vi "Send commands to tool.vi"(1 "Tool command":T1, 7 "Input Data":dbl, 11 "error in":errorcluster) -> (8 "OK":bool, 15 "error out":errorcluster)   [LabVIEW 2011]
uses:
  Stroker/def/Tool specific commands.ctl
  List of nodes in tool.ctl
  List of tools.ctl
  Variable List Tool Analog.ctl
  GUI/Controls/Slips Type Radio.ctl
  Application Structure/Loop ID.ctl
  emi Lib/System 01/0 - General/App/Loop control 2/Private/_emi_SMLoop Control Single.vi
  emi Lib/System 01/0 - General/App/Loop control/Private/_emi_GFV Loop Enable.vi
  emi Lib/System 01/0 - General/App/Loop control/Private/_emi_GFV Loop Linking.vi
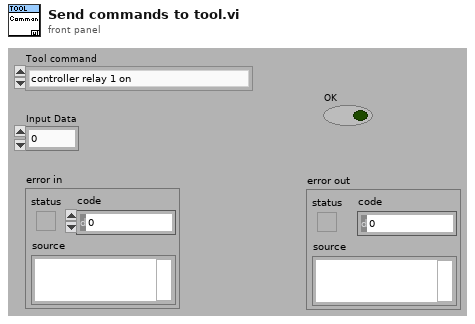
[diagram p1: front panel]
types:
  T1 = typedef "Tool specific commands.ctl" = enum16{"controller relay 1 on", "controller relay 1 off", "controller relay 2 on", "controller relay 2 off", "Solonoid 1 (master) on", "Solonoid 1 (master) off", "Solonoid 2 (Stroker) on", "Solonoid 2 (Stroker) off", "Solonoid 3 (Anchor) on", "Solonoid 3 (Anchor) off", "Controller relay 1 & 2 on", "Controller relay 1 & 2 off", "Controller relay 1 on, 2 off", "Controller relay 1 off, 2 on", "STROKER tool: Stop Force Mon", "High-G Stop", "High-G Get data", "High-G Stop Get data", "STROKER tool: Stroke out", "STROKER tool: Stroke in", "STROKER tool: Stroke stop", "STROKER tool: Stroke go to", "STROKER tool: Stop Homing", "STROKER tool: Start Force Mon dir in", "STROKER tool: Start Force Mon dir out", "Controller STOP"}
  T2 = typedef "List of tools.ctl" = enum16{"Stroker", "Driller", "Tractor"}
  T3 = typedef "Options  All pages and custom.ctl" = cluster{"P 1 (App)":T4, "P 2":T5, "P 3":T6, "P 4":T9, "P 5":T14, "P 6 (Err)":T15, "P 7 (Expert)":T16, "P 8 (Depth)":T18, "C 1":T19, "C 2":T20}
  T4 = typedef "Options Page 1 (App).ctl" = cluster{"Result files":path, "PCP Interface":string, "Tractor/Stroker Interface":string, "Tractor Interface":string, "Modem Status Interface":string, "Audible Alarm":bool, "Force alarm on Technical":bool, "Force alarm on HH":bool, "Force alarm on LL":bool, "Force alarm on H":bool, "Force alarm on L":bool}
  T5 = typedef "Options Page 2.ctl" = cluster{"Solenoid & Relay latching time":u16, "Tractor relay 1":dbl, "Tractor relay 2":dbl, "Tractor Solenoid limit":dbl}
  T6 = typedef "Options Page 3.ctl" = cluster{"Min resistance":dbl, "Max resistance":dbl, "Head voltage range":T7, "Max voltage jump":dbl, "Maximum resistance change":dbl, "Start Telemetry Voltage":dbl, "Start Telemetry Timeout":dbl, "Start Motor Voltage":dbl, "Stop Motor Voltage":dbl, "Pass Mode Warning Voltage":dbl, "Relay Switch Voltage":dbl, "Relay Status Loss Voltage":dbl, "Samples to average":i32, "PSU type DO NOT USE":T8, "Magna OVP":dbl, "Magna Current Limit":dbl}
  T7 = typedef "PCP type List.ctl" = enum16{"0 - 350V", "0 - 450V", "0 - 600V"}
  T8 = typedef "PSU Type.ctl" = enum16{"Unipower", "Magna 8.3A", "Magna 12A", "None"}
  T9 = typedef "Options Page 4.ctl" = cluster{"Solenoid & Relay latching time":u16, "Stroker relay 1":dbl, "Stroker Relay 2":dbl, "Stroker Solenoid limit":dbl, "Force det.":T10, "Stroke force lim.":dbl, "Anchor Enabled Pressure":dbl, "Tacometer puls":dbl, "Default anchor behavior":T11, "Default stroker behavior":T12, "Default stroker force limit (tonne)":dbl, "Slips Size":T13}
  T10 = typedef "Stroke force selector.ctl" = enum16{"Stroke in = node 1", "Strok out = node 1"}
  T11 = typedef "Default anchor behavior.ctl" = enum16{"Do nothing", "Set Anchor", "Release Anchor"}
  T12 = typedef "Default stroker behavior.ctl" = enum16{"Do nothing", "Stop", "Go Out", "Go In"}
  T13 = typedef "Slips Type Radio.ctl" = enum32{"No Selection", "338 MRS", "3,9 MRS"}
  T14 = typedef "Options Page 5.ctl" = cluster{"Solenoid & Relay latching time":u16, "Driller relay 1":dbl, "Driller Relay 2":dbl, "Driller  Solenoid limit":dbl}
  T15 = typedef "Options Page 6 (Err).ctl" = cluster{"Error and event files":path}
  T16 = typedef "Options Page 7 (Expert).ctl" = cluster{"Show Debug":bool, "Log debug messages":bool, "Additional debug messages":bool, "Start Beagle with Simulator data":bool, "Workshop mode":bool, "Modem baud":u16, "enumCANCOM":bool, "Modem sim":T17, "Telemetry Timeout Disable":i32, "Buffer size":i32, "Upd regular data":bool, "Cable comp":cluster{"VMOD1 Voltage(V)":dbl, "VMOD2 Voltage(V)":dbl}}
  T17 = typedef "Modem simulation setup.ctl" = cluster{"Modem dealay sim":bool, "Sim baud Tx":u16, "Bit Error fraction Tx":dbl, "Sim baud Rx":u16, "Bit Error fraction Rx":dbl}
  T18 = typedef "Options Page 8 (Depth).ctl" = cluster{"Winch Spool Circumference":dbl, "Winch Pulses per Revolution":dbl, "Current Depth":dbl}
  T19 = typedef "Options Custom 1.ctl" = cluster{"Depth Updated":bool, "Depth Offset":dbl}
  T20 = typedef "Options Custom 2.ctl" = cluster{"Placeholder":bool}
  T21 = typedef "Variable List Tool Analog.ctl" = enum16{"Tool Max Temperature", "Tool (Controller) Temperature", "Tool Supply Voltage", "Tool (Controller) Current", "Tool Acceleration X", "Tool Acceleration Y", "Tool Acceleration Z", "Tool Acceleration Sum", "Tool Inclination", "Tool Rotation", "Tool GP Sensor 1", "Tool GP Sensor 2", "Tool (Pressure 1) Temperature", "Tool Pressure 1 RAW", "Tool (Pressure 2) Temperature", "Tool Pressure 2 RAW", "Tool (Solenoid) Temperature", "Tool Solenoid Position", "PSU Temp", "Head Voltage", "PSU Main Voltage out", "PSU Main Current out", "Upper Tension Sub Temp", "Tool Upper Tension Sub Raw", "Lower Tension Sub Temp", "Tool Lower Tension Sub Raw", "Tool Var27 - Reserved", "Tool Var28 - Reserved", "Tool Var29 - Reserved", "Tool Var30 - Reserved", "Stroke Extension", "Stroke In Force", "Stroke Out Force", "Stroke Force", "Stroker Pressure 1", "Stroker Pressure 2", "Stroker Upper Tension Sub", "Stroker Lower Tension Sub", "Stroker Var09 - Reserved", "Stroker Var10 - Reserved", "Tractor Upper Tension Sub", "Tractor Lower Tension Sub", "Tractor Var03 - Reserved", "Tractor Var04 - Reserved", "Tool Temperature sensor", "Tool Motor Voltage", "Tool Motor Current", "Tool Motor Torque", "Tool weight on bit", "Tool Motor RPM"}
  T22 = typedef "Loop ID.ctl" = enum16{"Main-QSM", "Main-Dialog", "Main-Ind Upd", "Main-Graph Upd", "Main-Debug", "Main-DebugW1", "Main-DebugW2", "Main-SE Handler", "Interface-PCP", "Interface-CANbus", "Interface-Modem", "Var Handling-Beat", "Var Handling-From PCP", "Var Handling-File storage", "Var Handling-From Simulator", "GUI-GrphW Mast", "GUI-GrphW Slav", "SIM-Tool W1", "SIM-Tool W2", "Alm-Sound", "LEIN-motor", "Tool data gatherer Qer", "Tool Data LEIN STAT2 dekoder", "Indicator Value Update", "Tool STAT2 dedicated reader", "Tool ID handler", "Detail View L1", "Detail View L2", "Main display enable view", "Sequence runner", "Voltage setpoint", "Resistance setpoint", "Stroker Wizard L1", "Stroker Wizard L2", "Alarm Handling", "Annotations Tip Strip", "Magna Interface", "Modem Status", "Var Handling - Modem Status", "Power interface detector"}
  T23 = typedef "LEIN custom reply Q.ctl" = refnum<queue>
  T24 = typedef "List of nodes in tool.ctl" = u16
  T25 = typedef "User Setting Analog Channel Bg.ctl" = cluster{"Scaling":T26, "Limits and responces":T27, "Allow Graph selection by user":bool, "Unit":u16}
  T26 = typedef "Scaling.ctl" = cluster{"Gain":dbl, "Offset":dbl}
  T27 = typedef "Alarm Setup Analog.ctl" = cluster{"Technical Error(NA)":T28, "LL":T28, "L":T28, "H":T28, "HH":T28, "Limits":T30}
  T28 = typedef "Alarm Responce.ctl" = cluster{"Action":T29, "Alarm":bool}
  T29 = typedef "Action List.ctl" = enum16{"No Action", "Stop Motor", "Turn Off HV"}
  T30 = typedef "Limits.ctl" = cluster{"LL":dbl, "L":dbl, "H":dbl, "HH":dbl}
  T31 = typedef "LEIN Reply Holder.ctl" = cluster{"Reply msg(cmdif no reply)":T32, "Reply time":timestamp, "Valid reply":bool}
  T32 = typedef "LEIN CMD Cluster.ctl" = cluster{"SID":u8, "ANF":bool, "CMD":T33, "DATA":u8[]}
  T33 = typedef "LEIN CMD List.ctl" = enum8{"ACTI", "TASK", "RES0", "STAT", "RES1", "RES2", "RES3", "USER"}
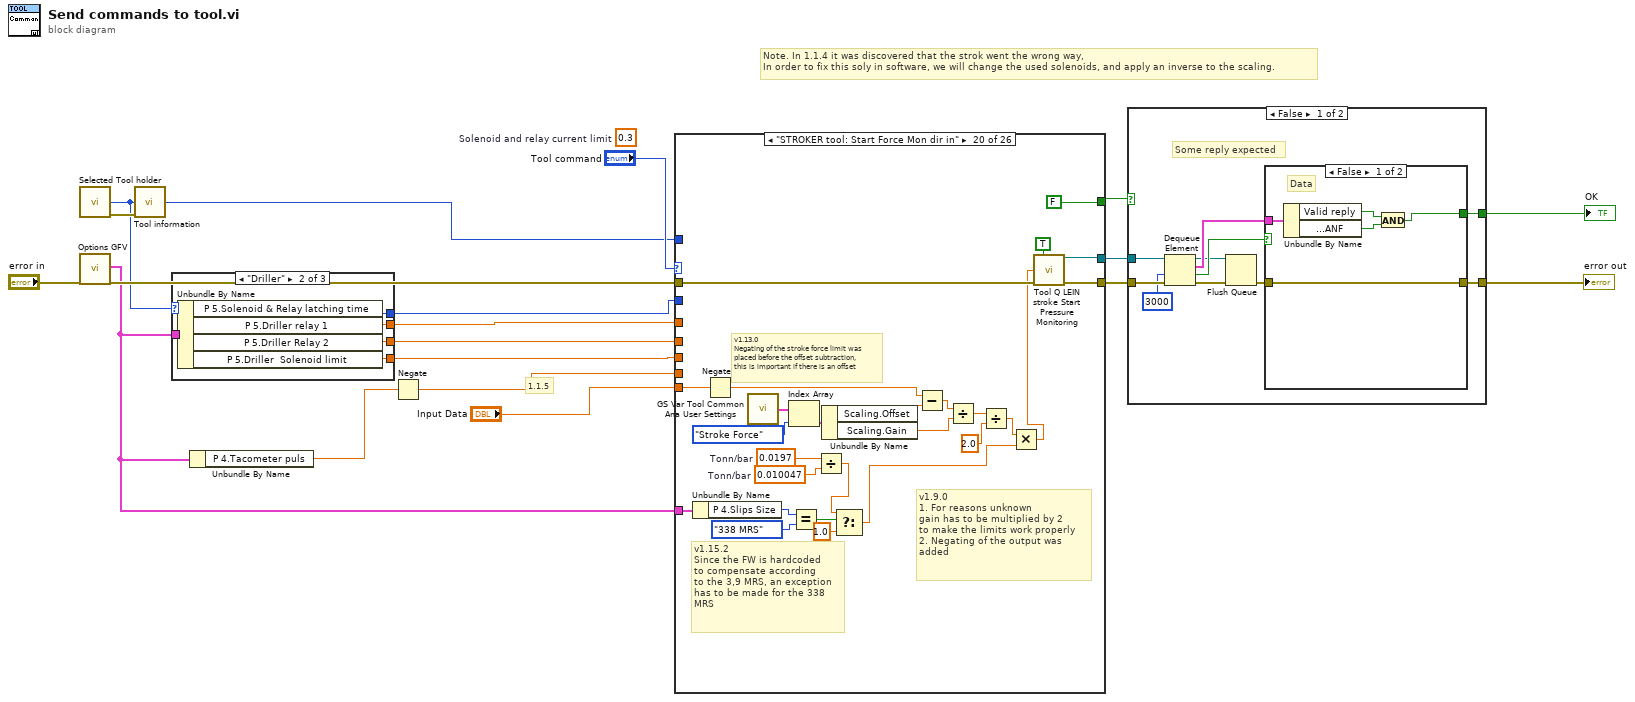
[diagram p0: block diagram]
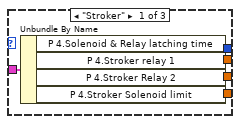
[diagram p2: hidden frame]
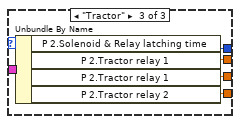
[diagram p3: hidden frame]
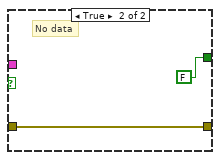
[diagram p4: hidden frame]
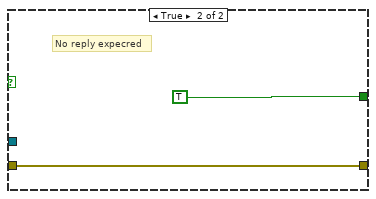
[diagram p5: hidden frame]
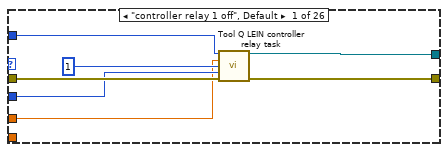
[diagram p6: hidden frame]
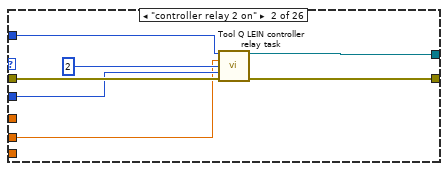
[diagram p7: hidden frame]
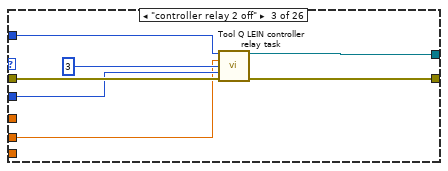
[diagram p8: hidden frame]
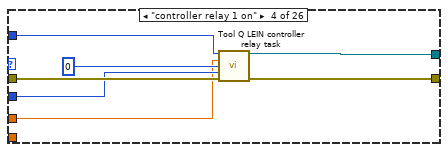
[diagram p9: hidden frame]
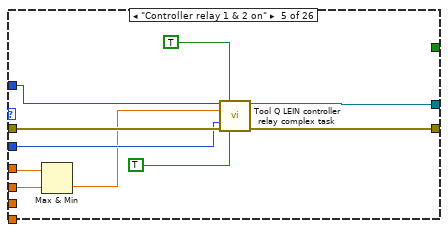
[diagram p10: hidden frame]
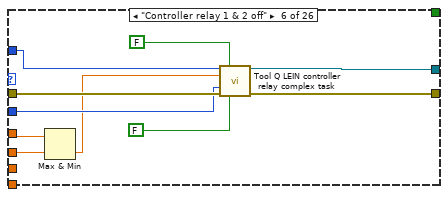
[diagram p11: hidden frame]
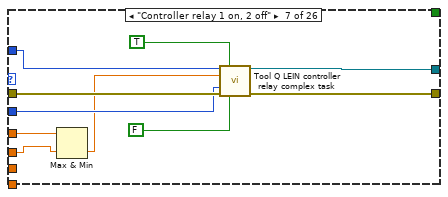
[diagram p12: hidden frame]
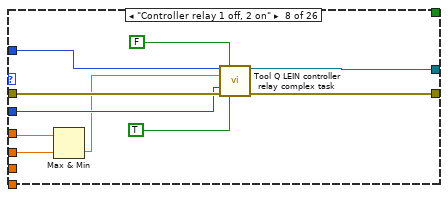
[diagram p13: hidden frame]
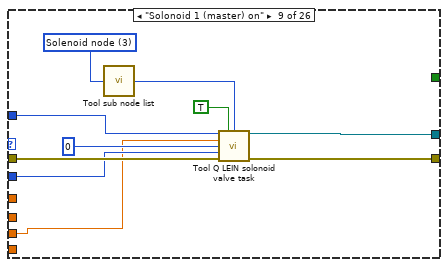
[diagram p14: hidden frame]
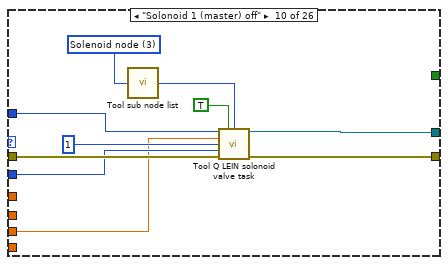
[diagram p15: hidden frame]
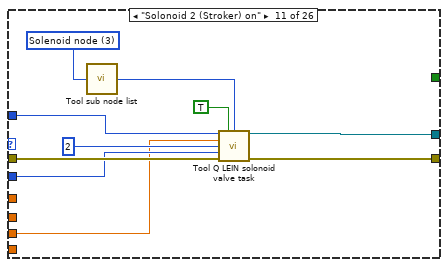
[diagram p16: hidden frame]
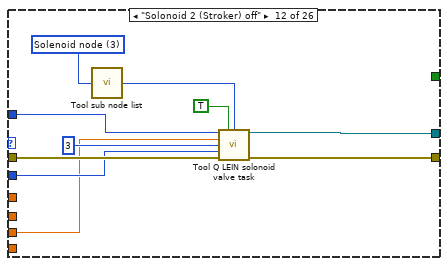
[diagram p17: hidden frame]
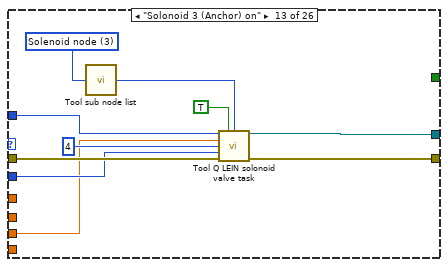
[diagram p18: hidden frame]
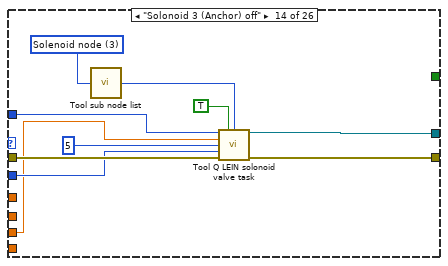
[diagram p19: hidden frame]
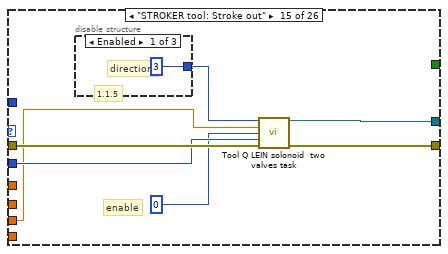
[diagram p20: hidden frame]
diagram:
  (unwired) 0.3  # Solenoid and relay current limit
  # "1.1.5"
  # "Note. In 1.1.4 it was discovered that the strok went the wrong way,\nIn order to fix this soly in software, we will change the used solenoids, and apply an inverse to the scaling."
  n1 = call "Selected Tool holder.vi"() -> ("Tool out"=w3:T2, "error out"=w6:errorcluster)  [unwired: 14 in]
  n2 = call "Options GFV.vi"("error in (no error)"="error in") -> ("Options"=w2:T3, "error out"=w11:errorcluster)  [unwired: 16 in, 1 out]
  n3 = call "Tool information.vi"("Tool in"=w3, "error in (no error)"=w6) -> ("Main node address"=w4:u8)  [unwired: 10 in, 3 out]
  n4 = case shown="\"Driller\"" w3 {
    tunnel: [w24 w29 w34] -> w10
    tunnel: [w23 w28 w33] -> w9
    tunnel: [w22 w27 w32] -> w8
    tunnel: w2 -> [w21 w26 w31]
    tunnel: [w20 w25 w30] -> w1
    frame "Stroker" {
      n5 = Unbundle By Name(w21) -> ("P 4.Solenoid & Relay latching time"=w20:u16, "P 4.Stroker relay 1"=w24:dbl, "P 4.Stroker Relay 2"=w23:dbl, "P 4.Stroker Solenoid limit"=w22:dbl)
    }
    frame "Driller" {
      n6 = Unbundle By Name(w26) -> ("P 5.Solenoid & Relay latching time"=w25:u16, "P 5.Driller relay 1"=w29:dbl, "P 5.Driller Relay 2"=w28:dbl, "P 5.Driller  Solenoid limit"=w27:dbl)
    }
    frame "Tractor" {
      n7 = Unbundle By Name(w31) -> ("P 2.Solenoid & Relay latching time"=w30:u16, "P 2.Tractor relay 1"=w34:dbl, "P 2.Tractor relay 1"=w33:dbl, "P 2.Tractor relay 2"=w32:dbl)
    }
  }
  n8 = Unbundle By Name(w2) -> ("P 4.Tacometer puls"=w5:dbl)
  n9 = Negate(x=w5) -> (-x=w7:dbl)
  n10 = case shown="\"STROKER tool: Start Force Mon dir in\"" "Tool command" {
    tunnel: [w40 w47 w54 w61 w70 w80 w90 w100 w111 w121 w131 w141 w151 w161 w169 w178 w187 w207 w212 w237 w261 w267 w281 w285 w290 w295] -> w16
    tunnel: w11 -> [w41 w48 w55 w62 w72 w82 w92 w102 w112 w122 w132 w142 w152 w162 w168 w177 w189 w208 w213 w238 w262 w268 w282 w286 w291 w296]
    tunnel: w1 -> [w39 w46 w53 w60 w71 w81 w91 w101 w110 w120 w130 w140 w150 w160 w167 w176 w188 w206 _ _ _ _ _ _ _ _]
    tunnel: "Input Data" -> [_ _ _ _ _ _ _ _ _ _ _ _ _ _ _ _ _ w196 _ w226 w254 _ _ _ _ _]
    tunnel: [w37 w44 w51 w58 w67 w77 w87 w97 w108 w118 w128 w138 w148 w158 w164 w173 w185 w205 w210 w235 w260 w266 w280 _ _ w294] -> w15
    tunnel: [_ _ _ _ _ _ _ _ _ _ _ _ _ _ _ _ _ _ FALSE FALSE FALSE _ _ TRUE TRUE _] -> w17
    tunnel: w10 -> [w36 _ _ w57 w65 w75 w86 w95 _ _ _ _ _ _ _ _ _ _ _ _ _ _ _ _ _ _]
    tunnel: w9 -> [_ w43 w50 _ w66 w76 w85 w96 _ _ _ _ _ _ _ _ _ _ _ _ _ _ _ _ _ _]
    tunnel: w8 -> [_ _ _ _ _ _ _ _ w106 w116 w126 w136 w146 w156 w163 w172 w184 w203 _ _ _ _ _ _ _ _]
    tunnel: w7 -> [_ _ _ _ _ _ _ _ _ _ _ _ _ _ _ _ _ w201 _ _ _ _ _ _ _ _]
    tunnel: w4 -> [w35 w42 w49 w56 w63 w73 w83 w93 w105 w115 w125 w135 w143 w155 _ _ _ _ _ _ _ w265 w279 _ _ w293]
    tunnel: w2 -> [_ _ _ _ _ _ _ _ _ _ _ _ _ _ _ _ _ _ _ w224 w243 _ _ _ _ _]
    frame "controller relay 1 off", Default {
      n11 = call "Tool Q LEIN controller relay task.vi"("Controller addres"=w35, "current limit(0.2A)"=w36, "outpuyt channel"=u8 1, "time (50 ms)"=w39, "error in (no error)"=w41) -> ("LEIN custom reply Q"=w37:T23, "error out"=w40:errorcluster)  [unwired: 9 in]
    }
    frame "controller relay 2 on" {
      n12 = call "Tool Q LEIN controller relay task.vi"("Controller addres"=w42, "current limit(0.2A)"=w43, "outpuyt channel"=u8 2, "time (50 ms)"=w46, "error in (no error)"=w48) -> ("LEIN custom reply Q"=w44:T23, "error out"=w47:errorcluster)  [unwired: 9 in]
    }
    frame "controller relay 2 off" {
      n13 = call "Tool Q LEIN controller relay task.vi"("Controller addres"=w49, "current limit(0.2A)"=w50, "outpuyt channel"=u8 3, "time (50 ms)"=w53, "error in (no error)"=w55) -> ("LEIN custom reply Q"=w51:T23, "error out"=w54:errorcluster)  [unwired: 9 in]
    }
    frame "controller relay 1 on" {
      n14 = call "Tool Q LEIN controller relay task.vi"("Controller addres"=w56, "current limit(0.2A)"=w57, "outpuyt channel"=u8 0, "time (50 ms)"=w60, "error in (no error)"=w62) -> ("LEIN custom reply Q"=w58:T23, "error out"=w61:errorcluster)  [unwired: 9 in]
    }
    frame "Controller relay 1 & 2 on" {
      n15 = Max & Min(x=w65, y=w66) -> (min(x,y)=w64:dbl)  [unwired: 1 out]
      n16 = call "Tool Q LEIN controller relay complex task.vi"("Controller ID"=w63, "Relay 1 close(on)"=TRUE, "current limit(0.2A)"=w64, "time (50 ms)"=w71, "error in (no error)"=w72, "Relay 2 close(on)"=TRUE) -> ("LEIN custom reply Q"=w67:T23, "error out"=w70:errorcluster)  [unwired: 8 in]
    }
    frame "Controller relay 1 & 2 off" {
      n17 = Max & Min(x=w75, y=w76) -> (min(x,y)=w74:dbl)  [unwired: 1 out]
      n18 = call "Tool Q LEIN controller relay complex task.vi"("Controller ID"=w73, "Relay 1 close(on)"=FALSE, "current limit(0.2A)"=w74, "time (50 ms)"=w81, "error in (no error)"=w82, "Relay 2 close(on)"=FALSE) -> ("LEIN custom reply Q"=w77:T23, "error out"=w80:errorcluster)  [unwired: 8 in]
    }
    frame "Controller relay 1 on, 2 off" {
      n19 = Max & Min(x=w86, y=w85) -> (min(x,y)=w84:dbl)  [unwired: 1 out]
      n20 = call "Tool Q LEIN controller relay complex task.vi"("Controller ID"=w83, "Relay 1 close(on)"=TRUE, "current limit(0.2A)"=w84, "time (50 ms)"=w91, "error in (no error)"=w92, "Relay 2 close(on)"=FALSE) -> ("LEIN custom reply Q"=w87:T23, "error out"=w90:errorcluster)  [unwired: 8 in]
    }
    frame "Controller relay 1 off, 2 on" {
      n21 = Max & Min(x=w95, y=w96) -> (min(x,y)=w94:dbl)  [unwired: 1 out]
      n22 = call "Tool Q LEIN controller relay complex task.vi"("Controller ID"=w93, "Relay 1 close(on)"=FALSE, "current limit(0.2A)"=w94, "time (50 ms)"=w101, "error in (no error)"=w102, "Relay 2 close(on)"=TRUE) -> ("LEIN custom reply Q"=w97:T23, "error out"=w100:errorcluster)  [unwired: 8 in]
    }
    frame "Solonoid 1 (master) on" {
      w104 = T24 3 items=["Main Controller", "Pressure node 1", "Pressure node 2", "Solenoid node"] ("Node")
      n23 = call "Tool sub node list.vi"("Tool node"=w104) -> ("SID"=w103:u8)  [unwired: 7 in, 7 out]
      n24 = call "Tool Q LEIN solonoid valve task.vi"("Main Controller ID"=w105, "Retry on err (F)"=TRUE, "Solonoid ID"=w103, "current limit(0.2A)"=w106, "outpuyt channel"=u8 0, "time (50 ms)"=w110, "error in (no error)"=w112) -> ("LEIN custom reply Q"=w108:T23, "error out"=w111:errorcluster)  [unwired: 7 in]
    }
    frame "Solonoid 1 (master) off" {
      w114 = T24 3 items=["Main Controller", "Pressure node 1", "Pressure node 2", "Solenoid node"] ("Node")
      n25 = call "Tool sub node list.vi"("Tool node"=w114) -> ("SID"=w113:u8)  [unwired: 7 in, 7 out]
      n26 = call "Tool Q LEIN solonoid valve task.vi"("Main Controller ID"=w115, "Retry on err (F)"=TRUE, "Solonoid ID"=w113, "current limit(0.2A)"=w116, "outpuyt channel"=u8 1, "time (50 ms)"=w120, "error in (no error)"=w122) -> ("LEIN custom reply Q"=w118:T23, "error out"=w121:errorcluster)  [unwired: 7 in]
    }
    frame "Solonoid 2 (Stroker) on" {
      w124 = T24 3 items=["Main Controller", "Pressure node 1", "Pressure node 2", "Solenoid node"] ("Node")
      n27 = call "Tool sub node list.vi"("Tool node"=w124) -> ("SID"=w123:u8)  [unwired: 7 in, 7 out]
      n28 = call "Tool Q LEIN solonoid valve task.vi"("Main Controller ID"=w125, "Retry on err (F)"=TRUE, "Solonoid ID"=w123, "current limit(0.2A)"=w126, "outpuyt channel"=u8 2, "time (50 ms)"=w130, "error in (no error)"=w132) -> ("LEIN custom reply Q"=w128:T23, "error out"=w131:errorcluster)  [unwired: 7 in]
    }
    frame "Solonoid 2 (Stroker) off" {
      w134 = T24 3 items=["Main Controller", "Pressure node 1", "Pressure node 2", "Solenoid node"] ("Node")
      n29 = call "Tool sub node list.vi"("Tool node"=w134) -> ("SID"=w133:u8)  [unwired: 7 in, 7 out]
      n30 = call "Tool Q LEIN solonoid valve task.vi"("Main Controller ID"=w135, "Retry on err (F)"=TRUE, "Solonoid ID"=w133, "current limit(0.2A)"=w136, "outpuyt channel"=u8 3, "time (50 ms)"=w140, "error in (no error)"=w142) -> ("LEIN custom reply Q"=w138:T23, "error out"=w141:errorcluster)  [unwired: 7 in]
    }
    frame "Solonoid 3 (Anchor) on" {
      w145 = T24 3 items=["Main Controller", "Pressure node 1", "Pressure node 2", "Solenoid node"] ("Node")
      n31 = call "Tool sub node list.vi"("Tool node"=w145) -> ("SID"=w144:u8)  [unwired: 7 in, 7 out]
      n32 = call "Tool Q LEIN solonoid valve task.vi"("Main Controller ID"=w143, "Retry on err (F)"=TRUE, "Solonoid ID"=w144, "current limit(0.2A)"=w146, "outpuyt channel"=u8 4, "time (50 ms)"=w150, "error in (no error)"=w152) -> ("LEIN custom reply Q"=w148:T23, "error out"=w151:errorcluster)  [unwired: 7 in]
    }
    frame "Solonoid 3 (Anchor) off" {
      w154 = T24 3 items=["Main Controller", "Pressure node 1", "Pressure node 2", "Solenoid node"] ("Node")
      n33 = call "Tool sub node list.vi"("Tool node"=w154) -> ("SID"=w153:u8)  [unwired: 7 in, 7 out]
      n34 = call "Tool Q LEIN solonoid valve task.vi"("Main Controller ID"=w155, "Retry on err (F)"=TRUE, "Solonoid ID"=w153, "current limit(0.2A)"=w156, "outpuyt channel"=u8 5, "time (50 ms)"=w160, "error in (no error)"=w162) -> ("LEIN custom reply Q"=w158:T23, "error out"=w161:errorcluster)  [unwired: 7 in]
    }
    frame "STROKER tool: Stroke out" {
      # "enable"
      n35 = disable-structure shown="Enabled" {
        disable-tunnel: [u8 3 ("outpuyt channel1") u8 2 ("outpuyt channel1") _] -> w166
        frame Enabled {
          # "1.1.5"
          # "direction"
        }
        frame Disabled {
          # "1.1.4"
          # "direction"
        }
        frame Disabled {
        }
      }
      n36 = call "Tool Q LEIN solonoid  two valves task.vi"("outpuyt channel1"=w166, "current limit(0.2A)"=w163, "outpuyt channel2"=u8 0, "time (50 ms)"=w167, "error in (no error)"=w168) -> ("LEIN custom reply Q"=w164:T23, "error out"=w169:errorcluster)  [unwired: 9 in]
    }
    frame "STROKER tool: Stroke in" {
      # "enable"
      n37 = disable-structure shown="Enabled" {
        disable-tunnel: [u8 2 ("outpuyt channel1") u8 3 ("outpuyt channel1") _] -> w175
        frame Enabled {
          # "1.1.5"
          # "direction"
        }
        frame Disabled {
          # "1.1.4"
          # "direction"
        }
        frame Disabled {
        }
      }
      n38 = call "Tool Q LEIN solonoid  two valves task.vi"("outpuyt channel1"=w175, "current limit(0.2A)"=w172, "outpuyt channel2"=u8 0, "time (50 ms)"=w176, "error in (no error)"=w177) -> ("LEIN custom reply Q"=w173:T23, "error out"=w178:errorcluster)  [unwired: 9 in]
    }
    frame "STROKER tool: Stroke stop" {
      n39 = call "Tool information.vi"("Tool in"=List_of_tools."Stroker") -> ("Main node address"=w182:u8)  [unwired: 11 in, 3 out]
      n40 = call "Tool Q LEIN solonoid valve task.vi"("Main Controller ID"=w182, "Retry on err (F)"=TRUE, "Solonoid ID"=u8 16, "current limit(0.2A)"=w184, "outpuyt channel"=u8 1, "time (50 ms)"=w188, "error in (no error)"=w189) -> ("LEIN custom reply Q"=w185:T23, "error out"=w187:errorcluster)  [unwired: 7 in]
    }
    frame "STROKER tool: Stroke go to" {
      # "v1.8.0 new unit system\n1. Convert to m which is the default unit\n2. Convert to mm which is used by hw\n3. Convert to pulses"
      # "1.1.5"
      n41 = call "GS Var Tool Common Ana User Settings.vi"() -> ("Tool Analog var User settigns out"=w199:T25[])  [unwired: 13 in, 2 out]
      n42 = Index Array(array=w199, index=Variable_List_Tool_Analog."Stroke Extension" ("Variable ID")) -> (element=w198:T25)
      n43 = Unbundle By Name(w198) -> ("Scaling.Offset"=w192:dbl, "Scaling.Gain"=w197:dbl)
      n44 = Subtract(x=w196, y=w192) -> (x-y=w200:dbl)
      n45 = Divide(x=w200, y=w197) -> (x/y=w194:dbl)
      n46 = Multiply(x=w194, y=1000.0) -> (x*y=w193:dbl)
      n47 = Multiply(x=w193, y=w201) -> (x*y=w202:dbl)
      n48 = call "Tool Q LEIN stroke Go To.vi"("Retry on err (F)"=TRUE, "current limit(0.2A)"=w203, "Target positio pulses"=w202, "time (50 ms)"=w206, "error in (no error)"=w208) -> ("LEIN custom reply Q"=w205:T23, "error out"=w207:errorcluster)  [unwired: 9 in]
    }
    frame "STROKER tool: Stop Homing" {
      n49 = call "Tool Q LEIN stroke Stop Homing.vi"("Retry on err (F)"=TRUE, "error in (no error)"=w213) -> ("LEIN custom reply Q"=w210:T23, "error out"=w212:errorcluster)  [unwired: 12 in]
    }
    frame "STROKER tool: Start Force Mon dir in" {
      w218 = 0.010047  # Tonn/bar
      w219 = 0.0197  # Tonn/bar
      # "v1.15.2\nSince the FW is hardcoded\nto compensate according \nto the 3,9 MRS, an exception\nhas to be made for the 338\nMRS"
      # "v1.13.0\nNegating of the stroke force limit was\nplaced before the offset subtraction, \nthis is important if there is an offset"
      # "v1.9.0 \n1. For reasons unknown \ngain has to be multiplied by 2\nto make the limits work properly\n2. Negating of the output was\nadded"
      n50 = Unbundle By Name(w224) -> ("P 4.Slips Size"=w223:T13)
      n51 = Negate(x=w226) -> (-x=w225:dbl)
      n52 = call "GS Var Tool Common Ana User Settings.vi"() -> ("Tool Analog var User settigns out"=w233:T25[])  [unwired: 13 in, 2 out]
      n53 = Index Array(array=w233, index=Variable_List_Tool_Analog."Stroke Force" ("Variable ID")) -> (element=w232:T25)
      n54 = Equal?(x=w223, y=Slips_Type_Radio."338 MRS" ("P 4.Slips Size")) -> (x = y?=w221:bool)
      n55 = Divide(x=w219, y=w218) -> (x/y=w217:dbl)
      n56 = Unbundle By Name(w232) -> ("Scaling.Offset"=w231:dbl, "Scaling.Gain"=w230:dbl)
      n57 = Select(t=w217, s=w221, f=1.0) -> (s? t:f=w214:dbl)
      n58 = Subtract(x=w225, y=w231) -> (x-y=w234:dbl)
      n59 = Divide(x=w234, y=w230) -> (x/y=w229:dbl)
      n60 = Divide(x=w229, y=2.0) -> (x/y=w216:dbl)
      n61 = Multiply(x=w216, y=w214) -> (x*y=w215:dbl)
      n62 = call "Tool Q LEIN stroke Start Pressure Monitoring.vi"("Retry on err (F)"=TRUE, "Input value"=w215, "error in (no error)"=w238) -> ("LEIN custom reply Q"=w235:T23, "error out"=w237:errorcluster)  [unwired: 11 in]
    }
    frame "STROKER tool: Start Force Mon dir out" {
      w245 = 0.010047  # Tonn/bar
      w246 = 0.0197  # Tonn/bar
      # "v1.15.2\nSince the FW is hardcoded\nto compensate according \nto the 3,9 MRS, an exception\nhas to be made for the 338\nMRS"
      # "v1.9.0 \n1. For reasons unknown \ngain has to be multiplied by 2\nto make the limits work properly\n2. Negating of the output was\nremoved"
      n63 = Unbundle By Name(w243) -> ("P 4.Slips Size"=w250:T13)
      n64 = call "GS Var Tool Common Ana User Settings.vi"() -> ("Tool Analog var User settigns out"=w258:T25[])  [unwired: 13 in, 2 out]
      n65 = Index Array(array=w258, index=Variable_List_Tool_Analog."Stroke Force" ("Variable ID")) -> (element=w257:T25)
      n66 = Equal?(x=w250, y=Slips_Type_Radio."338 MRS" ("P 4.Slips Size")) -> (x = y?=w248:bool)
      n67 = Unbundle By Name(w257) -> ("Scaling.Offset"=w256:dbl, "Scaling.Gain"=w255:dbl)
      n68 = Divide(x=w246, y=w245) -> (x/y=w244:dbl)
      n69 = Select(t=w244, s=w248, f=1.0) -> (s? t:f=w240:dbl)
      n70 = Subtract(x=w254, y=w256) -> (x-y=w259:dbl)
      n71 = Divide(x=w259, y=w255) -> (x/y=w252:dbl)
      n72 = Divide(x=w252, y=2.0) -> (x/y=w242:dbl)
      n73 = Multiply(x=w242, y=w240) -> (x*y=w241:dbl)
      n74 = call "Tool Q LEIN stroke Start Pressure Monitoring.vi"("Retry on err (F)"=TRUE, "Input value"=w241, "error in (no error)"=w262) -> ("LEIN custom reply Q"=w260:T23, "error out"=w261:errorcluster)  [unwired: 11 in]
    }
    frame "STROKER tool: Stop Force Mon" {
      n75 = disable-structure shown="Enabled" {
        disable-tunnel: w268 -> [w274 w278]
        disable-tunnel: [w273 w277] -> w267
        disable-tunnel: [w270 w276] -> w266
        disable-tunnel: w265 -> [w269 _]
        frame Disabled {
          # "command for High-G Start - has been replaced\nwith stop force monitoring"
          n76 = call "Tool Q LEIN High G  Start.vi"("Controller ID"=w269, "G trigger limit(5 G)"=50.0, "Numb pre samples(250)"=u16 1000, "error in (no error)"=w274) -> ("LEIN custom reply Q"=w270:T23, "error out"=w273:errorcluster)  [unwired: 10 in]
        }
        frame Enabled {
          n77 = call "Tool Q LEIN stroke Stop Pressure Monitoring.vi"("Retry on err (F)"=TRUE, "error in (no error)"=w278) -> ("LEIN custom reply Q"=w276:T23, "error out"=w277:errorcluster)  [unwired: 12 in]
        }
      }
    }
    frame "High-G Stop" {
      n78 = call "Tool Q LEIN High G Stopp.vi"("Controller ID"=w279, "error in (no error)"=w282) -> ("LEIN custom reply Q"=w280:T23, "error out"=w281:errorcluster)  [unwired: 12 in]
    }
    frame "High-G Get data" {
      n79 = call-poly "emi_SMLoop Control.vi"("Loop ID in"=Loop_ID."Indicator Value Update" ("Loop ID"), "Enable"=TRUE, "error in (no error)"=w286) -> ("error out"=w285:errorcluster)  [unwired: 11 in, 1 out]
    }
    frame "High-G Stop Get data" {
      n80 = call-poly "emi_SMLoop Control.vi"("Loop ID in"=Loop_ID."Indicator Value Update" ("Loop ID"), "Enable"=FALSE, "error in (no error)"=w291) -> ("error out"=w290:errorcluster)  [unwired: 11 in, 1 out]
    }
    frame "Controller STOP" {
      n81 = call "LEIN CMD send ACTI 01 STOP.vi"("Controller"=w293, "Retry on err (F)"=TRUE, "error in (no error)"=w296) -> ("LEIN custom reply Q"=w294:T23, "error out"=w295:errorcluster)  [unwired: 11 in]
    }
  }
  n82 = case shown="False" w17 {
    tunnel: w16 -> [w307 w316]
    tunnel: [w304 w316] -> w13
    tunnel: w15 -> [w306 _]
    tunnel: [w303 TRUE ("Valid reply")] -> w14
    frame False {
      # "Some reply expected"
      n83 = Dequeue Element(queue=w306, timeout in ms (-1)=3000, error in (no error)=w307) -> (queue out=w298:T23, element=w302:T31, timed out?=w301:bool, error out=w299:errorcluster)
      n84 = Flush Queue(queue=w298, error in (no error)=w299) -> (error out=w300:errorcluster)  [unwired: 2 out]
      n85 = case shown="False" w301 {
        tunnel: w300 -> [w311 w314]
        tunnel: [w311 w314] -> w304
        tunnel: [w308 FALSE] -> w303
        tunnel: w302 -> [w312 _]
        frame False {
          # "Data"
          n86 = Unbundle By Name(w312) -> ("Valid reply"=w309:bool, "Reply msg(cmdif no reply).ANF"=w310:bool)
          n87 = And(x=w309, y=w310) -> (x .and. y?=w308:bool)
        }
        frame True {
          # "No data"
        }
      }
    }
    frame True {
      # "No reply expecred"
    }
  }
  "error out" <- w13
  "OK" <- w14
